vi "check_boundary.vi"(0 "vector x":dbl, 1 "vector y":dbl, 2 "position x":dbl, 3 "position y":dbl, 4 "speed":dbl, 5 "radius":dbl, 6 "player width":dbl, 7 "player left position y":dbl, 8 "player height":dbl, 9 "player right position y":dbl, 10 "window width":dbl, 11 "pause":dbl, 12 "window height":dbl) -> (14 "output vector x":dbl, 15 "output vector y":dbl, 16 "output x":dbl, 17 "output y":dbl, 18 "left win":i32, 19 "right win":i32)   [LabVIEW 2023]
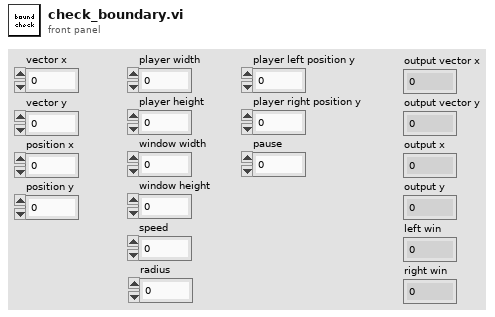
[diagram p1: front panel]
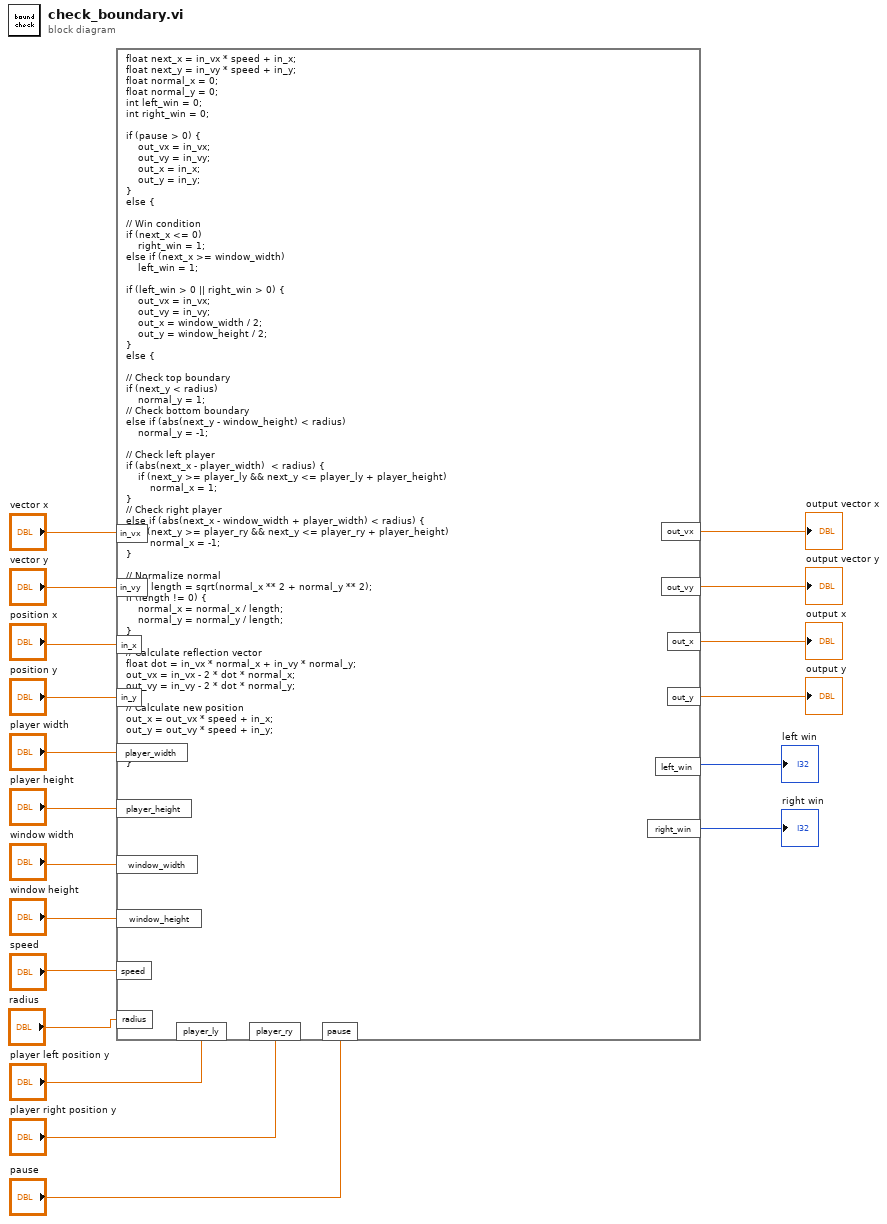
[diagram p0: block diagram]
diagram:
  # "power operator **"
  n1 = formula code="float next_x = in_vx * speed + in_x;\nfloat next_y = in_vy * speed + in_y;\nfloat normal_x = 0;\nfloat normal_y = 0;\nint left_win = 0;\nint right_win = 0;\n\nif (pause > 0) {\n    out_vx = in_vx;\n    out_vy = in_vy;\n    out_x = in_x;\n    out_y = in_y;\n}\nelse {\n\n// Win condition\nif (next_x <= 0) \n    right_win = 1;\nelse if (next_x >= window_width)\n    left_win = 1;\n\nif (left_win > 0 || right_win > 0) {\n    out_vx = in_vx;\n    out_vy = in_vy;\n    out_x = window_width / 2;\n    out_y = window_height / 2;\n}\nelse {\n\n// Check top boundary\nif (next_y < radius)\n    normal_y = 1;\n// Check bottom boundary\nelse if (abs(next_y - window_height) < radius)\n    normal_y = -1;\n\n// Check left player\nif (abs(next_x - player_width)  < radius) {\n    if (next_y >= player_ly && next_y <= player_ly + player_height)\n        normal_x = 1;\n}\n// Check right player\nelse if (abs(next_x - window_width + player_width) < radius) {\n    if (next_y >= player_ry && next_y <= player_ry + player_height)\n        normal_x = -1;\n}\n\n// Normalize normal\nfloat length = sqrt(normal_x ** 2 + normal_y ** 2);\nif (length != 0) {\n    normal_x = normal_x / length;\n    normal_y = normal_y / length;\n}\n\n// Calculate reflection vector\nfloat dot = in_vx * normal_x + in_vy * normal_y;\nout_vx = in_vx - 2 * dot * normal_x;\nout_vy = in_vy - 2 * dot * normal_y;\n\n// Calculate new position\nout_x = out_vx * speed + in_x;\nout_y = out_vy * speed + in_y;\n\n}\n}"("in_vx"="vector x", "in_vy"="vector y", "in_x"="position x", "in_y"="position y", "player_width"="player width", "window_width"="window width", "window_height"="window height", "speed"="speed", "player_height"="player height", "player_ly"="player left position y", "player_ry"="player right position y", "radius"="radius", "pause"="pause") -> ("out_vx"=→"output vector x":dbl, "out_vy"=→"output vector y":dbl, "out_x"=→"output x":dbl, "out_y"=→"output y":dbl, "left_win"=→"left win":i32, "right_win"=→"right win":i32)
